vi "niFpgaLRMRefOutSettingTemplate.vi"(0 "Name Control Type Specifier":string) -> (4 "ref out":string)   [LabVIEW 2017]
uses:
  <vilib>/rvi/DataTransferAndStorage/Container/Common/niFpgaContainerMetaDataKey.ctl
  <vilib>/rvi/DataTransferAndStorage/Container/Common/niFpgaContainerState.ctl
  <vilib>/rvi/DataTransferAndStorage/Container/Common/niFpgaDataTypeControl.ctl
  <vilib>/rvi/DataTransferAndStorage/Container/Common/niFpgaContainerImplementationControl.ctl
  <vilib>/rvi/DataTransferAndStorage/Container/Common/niFpgaContainerArbitrationOptionsControl.ctl
  <vilib>/rvi/DataTransferAndStorage/Container/Common/niFpgaTransferTypeControl.ctl
  <vilib>/rvi/DataTransferAndStorage/Container/Common/niFpgaContainerInitializationParameters.ctl
  <vilib>/rvi/Memory/Memory_Types/niFpgaMemoryInterfaceConfiguration.ctl
  <vilib>/rvi/FIFO/Fifo_Types/niFpgaFifoControlLogicControl.ctl
  <vilib>/rvi/DataTransferAndStorage/Container/Common/niFpgaContainerMemoryLatencyControl.ctl
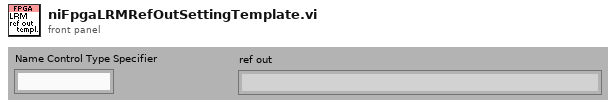
[diagram p1: front panel]
types:
  T1 = typedef "niFpgaContainerState.ctl" = cluster{"displayName":string, "hardwareName":string, "dataType":T2, "elementTypeDescriptor":variant, "terminalTypeDescriptor":variant, "requestedNumberOfElements":u32, "memoryType":T3, "arbitrationForInterfaceA":T4, "numberOfElementsPerRead":u32, "arbitrationForInterfaceB":T4, "numberOfElementsPerWrite":u32, "VI_Defined":bool, "type":T5, "initializationParameters":T6, "disableOnOverflow/Underflow":bool, "interfaceConfiguration":T7, "controlLogic":T8, "actualNumberOfElements":u32, "dramSelection":string, "dramMaxOustandingRequests":i32, "dramIncludeByteEnables":bool, "dramGrantTime":u32, "fullEmulation":bool, "memoryInMultipleClockDomains":bool, "memoryLatency":T9}
  T2 = typedef "niFpgaDataTypeControl.ctl" = enum32{"Boolean", "I8", "I16", "I32", "I64", "U8", "U16", "U32", "U64", "FXP", "CustomControl", "SGL"}
  T3 = typedef "niFpgaContainerImplementationControl.ctl" = enum16{"Flip-Flops", "Look-Up Table", "Block Memory", "DRAM"}
  T4 = typedef "niFpgaContainerArbitrationOptionsControl.ctl" = enum16{"Always Arbitrate", "Arbitrate if Multiple Requestors Only", "Never Arbitrate"}
  T5 = typedef "niFpgaTransferTypeControl.ctl" = enum16{"Target-Scoped", "Host to Target - DMA", "Target to Host - DMA", "Peer to Peer Reader", "Peer to Peer Writer", "Bidirectional"}
  T6 = typedef "niFpgaContainerInitializationParameters.ctl" = cluster{"initialized":bool, "VI_Path":path, "initialData":variant}
  T7 = typedef "niFpgaMemoryInterfaceConfiguration.ctl" = enum16{"Read A-Write B", "Read A-Read B"}
  T8 = typedef "niFpgaFifoControlLogicControl.ctl" = enum16{"Slice Fabric", "Target Optimal", "Built-in"}
  T9 = typedef "niFpgaContainerMemoryLatencyControl.ctl" = u16
  T10 = typedef "niFpgaContainerMetaDataKey.ctl" = enum16{"FPGA FIFO", "FPGA Memory", "FPGA Register", "FPGA Handshake"}
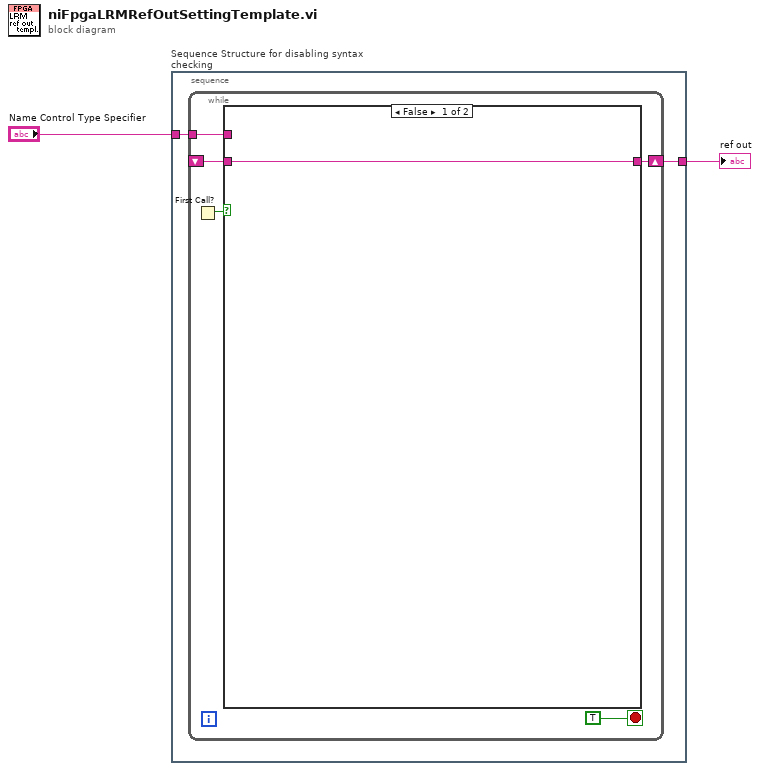
[diagram p0: block diagram]
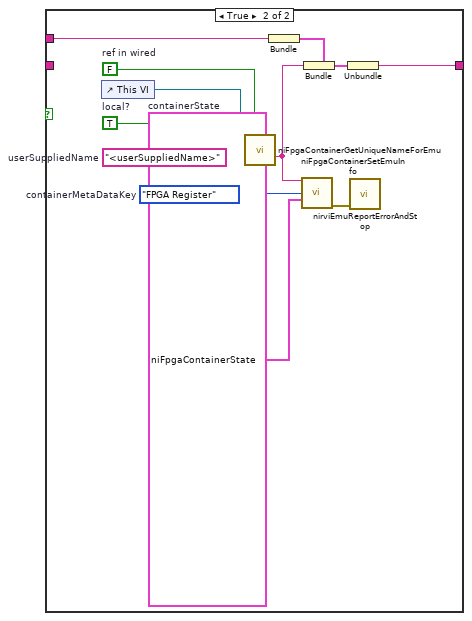
[diagram p2: hidden frame]
diagram:
  n1 = stacked-sequence "Sequence Structure for disabling syntax checking" {
    tunnel: "Name Control Type Specifier" -> [w3]
    tunnel: [w4] -> w1
    frame #0 {
      n2 = while {
        shift-right: [w9] -> w4
        shift-left: _ -> [w5]
        tunnel: w3 -> [w6]
        stop <- TRUE stop-if-true
        n3 = First Call?() -> (First Call?: T/F=w8:bool)
        n4 = case shown="False" w8 {
          tunnel: w6 -> [_ w22]
          tunnel: [w10 w19] -> w9
          tunnel: w5 -> [w10 _]
          frame False {
          }
          frame True {
            w11 = FALSE  # ref in wired
            w14 = TRUE  # local?
            w17 = T1 {"displayName"="", "hardwareName"="", "dataType"=enum."Boolean", "elementTypeDescriptor"=variant, "terminalTypeDescriptor"=variant, "requestedNumberOfElements"=0, "memoryType"=enum."Flip-Flops", "arbitrationForInterfaceA"=enum."Always Arbitrate", "numberOfElementsPerRead"=0, "arbitrationForInterfaceB"=enum."Always Arbitrate", "numberOfElementsPerWrite"=0, "VI_Defined"=FALSE, "type"=enum."Target-Scoped", "initializationParameters"={"initialized"=FALSE, "VI_Path"=path "", "initialData"=variant}, "disableOnOverflow/Underflow"=FALSE, "interfaceConfiguration"=enum."Read A-Write B", "controlLogic"=enum."Slice Fabric", "actualNumberOfElements"=0, "dramSelection"="", "dramMaxOustandingRequests"=0, "dramIncludeByteEnables"=FALSE, "dramGrantTime"=0, "fullEmulation"=FALSE, "memoryInMultipleClockDomains"=FALSE, "memoryLatency"=1}  # containerState
            w16 = niFpgaContainerMetaDataKey."FPGA Register"  # containerMetaDataKey
            w13 = "<userSuppliedName>"  # userSuppliedName
            n5 = control-ref of="This VI"() -> (w15:refnum<vi>)
            n6 = call <vilib>:"niFpgaContainerGetUniqueNameForEmu.vi"("parent VI"=w15, "ref in wired"=w11, "local"=w14, "name in"=w13) -> ("name out"=w12:string)  [unwired: 11 in]
            n7 = Bundle("Name Control Type Specifier"=w22) -> (w21:cluster{"Name Control Type Specifier":string})  [unwired: 1 in]
            n8 = call <vilib>:"niFpgaContainerSetEmuInfo.vi"("qualified name"=w12, "metaDataKey"=w16, "containerState"=w17) -> ("error out"=w18:errorcluster)  [unwired: 2 in, 10 out]
            n9 = Bundle(cluster=w21, "Name Control Type Specifier"=w12) -> (w20:cluster{"Name Control Type Specifier":string})
            n10 = Unbundle(w20) -> ("Name Control Type Specifier"=w19:string)
            n11 = call <vilib>:"nirviEmuReportErrorAndStop.vi"("error to report"=w18) -> ()  [unwired: 1 in, 14 out]
          }
        }
      }
    }
  }
  "ref out" <- w1
